vi "4-1.vi"() -> ()   [LabVIEW 2019, in "AoC2022.lvlib"]
uses:
  AoC2022.lvlib
panel:
  out "Array":string[](array[string])
  out "Numeric":i32
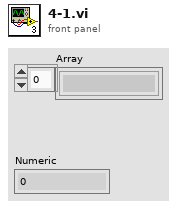
[diagram p1: front panel]
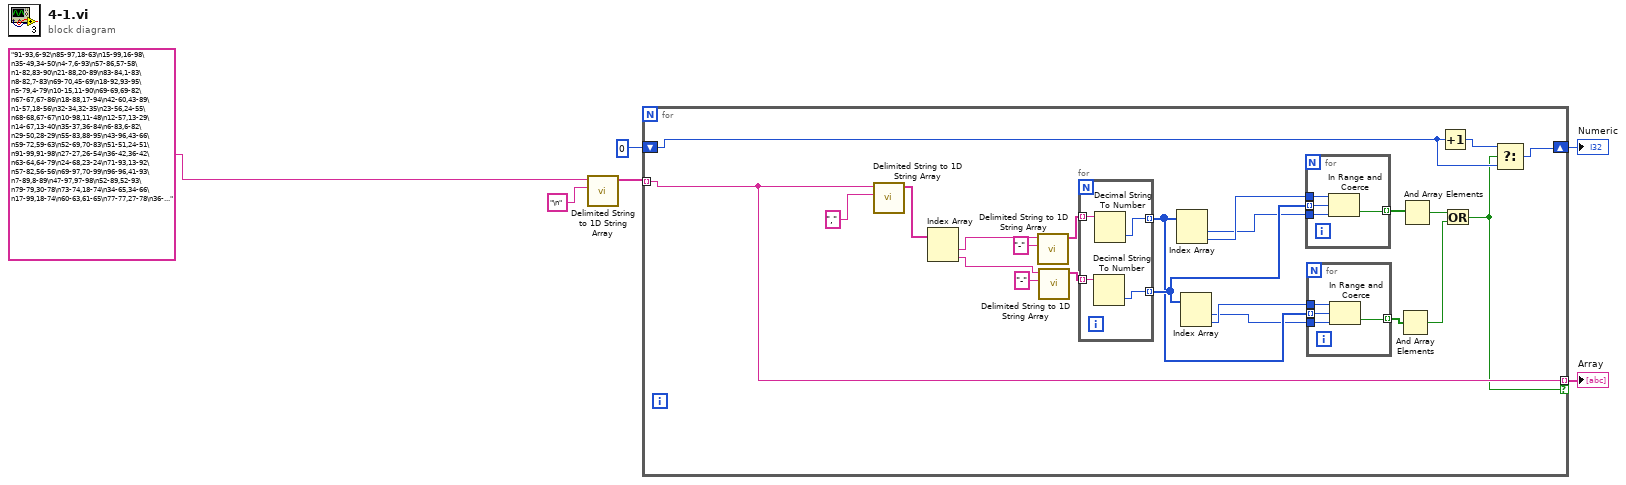
[diagram p0: block diagram]
diagram:
  n1 = call <vilib>:"Delimited String to 1D String Array.vi"("delimiter"="\n", "delimited string"="91-93,6-92\n85-97,18-63\n15-99,16-98\n35-49,34-50\n4-7,6-93\n57-86,57-58\n1-82,83-90\n21-88,20-89\n83-84,1-83\n8-82,7-83\n69-70,45-69\n18-92,93-95\n5-79,4-79\n10-15,11-90\n69-69,69-82\n67-67,67-86\n18-88,17-94\n42-60,43-89\n1-57,18-56\n32-34,32-35\n23-56,24-55\n68-68,67-67\n10-98,11-48\n12-57,13-29\n14-67,13-40\n35-37,36-84\n6-83,6-82\n29-50,28-29\n55-83,88-95\n43-96,43-66\n59-72,59-63\n52-69,70-83\n51-51,24-51\n91-99,91-98\n27-27,26-54\n36-42,36-42\n63-64,64-79\n24-68,23-24\n71-93,13-92\n57-82,56-56\n69-97,70-99\n96-96,41-93\n7-89,8-89\n47-97,97-98\n52-89,52-93\n79-79,30-78\n73-74,18-74\n34-65,34-66\n17-99,18-74\n60-63,61-65\n77-77,27-78\n36-52,51-53\n6-7,7-98\n14-35,36-91\n3-3,5-82\n24-24,25-97\n4-65,3-18\n2-9,10-90\n14-82,15-76\n3-3,3-32\n43-85,43-86\n91-91,23-92\n65-98,10-84\n8-71,9-72\n94-94,6-95\n64-66,65-65\n5-75,4-4\n19-76,20-55\n31-98,32-99\n3-83,3-12\n70-71,21-71\n28-36,37-50\n6-95,5-94\n56-56,56-67\n17-77,25-95\n24-50,25-51\n36-60,60-73\n30-50,48-63\n4-98,5-97\n42-42,42-56\n15-17,16-46\n35-69,36-70\n22-49,22-95\n41-77,36-36\n48-92,47-96\n7-89,6-88\n20-94,20-94\n9-75,73-76\n35-60,35-58\n35-90,35-94\n1-93,1-94\n26-26,26-45\n29-98,28-94\n55-86,45-68\n24-87,25-87\n94-94,17-93\n35-93,36-92\n9-28,9-90\n25-74,26-73\n12-79,11-98\n58-92,57-93\n1-64,2-63\n96-97,7-97\n44-62,62-69\n77-90,6-52\n1-96,96-97\n55-66,54-68\n1-86,1-85\n28-91,28-94\n6-89,5-89\n9-35,9-9\n2-22,1-34\n16-56,54-57\n36-44,44-68\n29-87,11-87\n30-32,31-54\n18-76,10-10\n12-13,13-26\n18-46,17-55\n12-53,13-54\n30-67,31-66\n22-60,22-22\n42-94,42-42\n6-65,66-98\n41-43,42-98\n47-71,48-72\n8-65,7-46\n25-63,6-12\n57-62,24-56\n15-29,14-33\n21-65,20-94\n27-94,28-89\n88-95,5-72\n65-80,64-81\n72-73,39-72\n22-48,21-48\n5-6,13-80\n54-80,55-79\n34-66,31-43\n26-52,51-66\n27-28,15-27\n90-99,89-99\n25-55,26-27\n29-94,29-95\n27-96,96-96\n35-65,65-66\n15-56,63-84\n36-83,35-37\n15-72,15-15\n14-90,15-34\n2-41,4-42\n48-75,47-56\n23-63,63-78\n8-90,5-89\n41-65,12-66\n48-61,54-60\n28-90,29-35\n51-83,85-87\n9-95,9-92\n57-76,57-69\n2-66,2-65\n7-92,11-92\n26-89,88-88\n37-37,37-86\n33-37,36-84\n3-97,99-99\n29-32,29-57\n35-69,5-35\n5-97,5-97\n60-86,44-87\n41-88,98-98\n52-55,53-57\n27-93,28-92\n95-97,50-91\n45-62,45-84\n1-60,2-42\n7-97,98-99\n91-92,18-91\n10-53,11-95\n75-80,77-84\n1-1,1-99\n7-77,27-41\n6-96,96-96\n17-97,17-96\n1-1,1-99\n28-90,29-32\n2-79,12-80\n47-47,10-46\n97-98,2-97\n38-64,38-40\n5-97,4-30\n8-91,7-92\n21-49,20-21\n21-77,20-95\n16-70,15-26\n33-98,32-96\n3-4,8-72\n48-98,2-99\n7-30,8-30\n34-60,33-34\n78-92,34-83\n5-46,5-5\n52-73,35-74\n37-96,97-99\n6-92,5-92\n3-85,3-84\n2-86,2-2\n93-98,72-92\n23-34,22-34\n6-73,5-7\n29-42,29-67\n12-97,11-29\n38-68,38-67\n85-87,81-86\n23-29,30-64\n2-3,3-83\n17-92,18-64\n28-29,29-38\n52-54,53-83\n6-19,6-90\n8-97,79-97\n2-40,2-30\n3-89,4-98\n6-89,1-3\n8-8,8-94\n5-94,4-93\n81-95,81-87\n86-88,87-89\n8-8,9-94\n46-56,46-46\n7-95,32-99\n3-93,2-31\n80-80,1-79\n64-98,63-64\n82-84,14-83\n26-79,26-80\n30-56,57-88\n6-15,49-93\n8-30,4-33\n55-99,13-97\n5-6,6-38\n10-49,12-50\n5-79,78-79\n7-93,6-94\n12-65,64-65\n14-15,15-90\n95-95,48-94\n1-93,3-94\n49-88,88-95\n13-13,13-83\n8-98,97-98\n20-22,21-43\n83-88,84-87\n22-88,21-88\n47-98,35-46\n1-5,6-82\n59-86,65-85\n38-43,40-64\n23-96,22-97\n81-83,67-80\n70-96,70-70\n72-89,62-67\n5-83,6-84\n10-85,2-15\n1-3,2-56\n2-37,37-38\n5-94,4-85\n1-2,3-97\n1-95,97-97\n14-29,15-20\n16-22,29-97\n80-89,89-90\n22-75,21-75\n9-88,6-7\n6-10,11-22\n9-79,9-80\n42-57,18-41\n34-96,96-97\n16-96,17-95\n21-21,22-85\n16-67,15-16\n23-72,60-71\n9-81,9-81\n44-91,45-92\n3-91,4-92\n38-92,69-91\n72-96,2-73\n2-46,1-85\n28-71,28-71\n8-81,7-9\n1-12,1-2\n10-92,3-91\n55-95,96-98\n40-50,41-98\n7-8,8-29\n22-48,23-61\n81-90,25-82\n17-34,17-72\n88-88,5-88\n34-78,34-77\n66-68,67-76\n50-98,49-50\n60-73,6-59\n12-71,12-70\n14-69,68-69\n5-7,6-79\n21-81,21-21\n3-30,4-29\n4-4,6-94\n20-85,19-20\n21-40,22-39\n3-93,2-93\n47-50,50-68\n4-97,5-99\n28-46,27-53\n18-18,17-86\n12-76,77-77\n10-96,11-78\n6-88,4-89\n7-98,7-98\n4-47,3-4\n37-41,38-61\n26-92,26-57\n8-49,14-50\n19-73,18-64\n70-71,3-70\n4-4,4-99\n11-99,62-74\n4-27,4-9\n38-65,38-66\n73-81,79-96\n11-75,10-10\n24-56,55-55\n30-30,31-75\n48-94,49-95\n2-98,3-8\n63-87,62-87\n7-95,73-97\n96-97,15-98\n8-58,57-64\n6-81,80-99\n34-78,78-79\n43-44,44-60\n68-78,78-78\n1-1,3-92\n30-57,53-56\n26-82,26-81\n24-92,24-91\n42-62,43-57\n28-76,77-85\n6-50,6-50\n8-70,9-86\n79-79,32-78\n21-93,27-94\n71-85,65-70\n40-85,41-73\n46-46,47-91\n3-99,4-98\n14-24,13-57\n11-15,17-82\n49-63,39-53\n26-27,19-26\n19-98,18-47\n3-96,3-3\n17-20,16-63\n2-14,2-27\n16-37,13-15\n13-14,14-84\n4-80,3-79\n15-79,14-15\n7-7,8-72\n12-99,99-99\n23-93,24-32\n4-26,3-58\n33-33,38-58\n60-75,59-61\n6-6,6-97\n3-34,2-95\n66-85,66-84\n8-65,9-40\n57-58,58-61\n4-41,5-28\n36-96,35-95\n5-94,1-95\n54-57,56-75\n26-26,26-41\n7-92,7-95\n26-33,5-32\n37-49,38-67\n42-51,52-55\n55-55,31-54\n1-1,1-32\n85-98,9-96\n97-97,77-96\n7-77,6-83\n73-89,72-95\n24-78,27-79\n8-14,3-7\n23-23,23-74\n4-74,3-73\n15-15,17-48\n3-99,3-3\n15-62,15-62\n21-97,6-37\n98-99,64-92\n40-65,41-58\n61-86,1-60\n95-96,23-95\n40-65,39-66\n3-66,2-4\n5-85,6-96\n86-88,85-89\n6-94,82-93\n31-31,32-75\n4-4,3-55\n18-83,19-84\n12-99,11-12\n51-53,49-54\n17-17,18-87\n4-62,61-61\n10-14,14-73\n5-78,6-79\n21-53,22-62\n37-39,38-39\n22-23,23-78\n31-83,35-84\n35-76,36-60\n67-69,68-82\n4-64,29-79\n42-43,52-87\n11-13,12-34\n25-65,70-71\n46-46,46-46\n5-80,3-55\n12-46,10-47\n16-49,1-16\n56-98,32-56\n36-83,37-99\n58-58,53-89\n66-74,8-48\n71-90,34-65\n10-79,1-3\n3-13,4-12\n65-66,66-99\n6-93,5-98\n17-90,18-40\n94-96,15-75\n83-90,99-99\n9-47,10-89\n5-79,6-81\n22-44,16-18\n7-7,7-90\n2-94,1-94\n33-68,24-34\n1-8,12-72\n87-96,73-93\n8-97,97-99\n18-45,19-46\n14-93,13-90\n47-47,48-48\n10-89,11-44\n43-75,76-94\n18-54,17-17\n6-82,7-84\n40-78,78-83\n15-15,16-21\n19-68,50-67\n25-27,30-77\n11-69,10-68\n38-38,48-84\n69-98,68-93\n11-16,17-93\n7-26,27-75\n73-97,73-93\n9-92,8-93\n23-62,62-99\n19-89,19-95\n51-53,15-52\n6-31,30-32\n93-94,10-49\n31-52,30-38\n43-45,44-92\n14-42,13-29\n21-24,22-80\n70-79,24-80\n49-49,49-87\n2-3,2-50\n5-95,6-95\n20-57,16-66\n38-69,68-68\n60-90,91-92\n55-97,94-99\n30-90,30-84\n29-51,30-51\n55-55,42-56\n9-96,8-97\n58-96,58-58\n37-97,98-99\n5-69,5-47\n20-93,21-84\n9-65,1-2\n23-24,24-69\n7-95,8-94\n7-43,8-99\n7-63,4-5\n4-17,4-21\n21-28,27-84\n10-23,10-88\n4-52,4-52\n99-99,89-97\n84-90,1-85\n51-90,99-99\n33-67,53-79\n29-29,2-30\n2-88,1-86\n16-99,3-98\n83-96,82-83\n83-85,20-84\n6-6,7-62\n44-78,58-94\n7-25,7-25\n7-94,8-80\n16-97,15-98\n4-52,51-71\n75-92,49-69\n2-94,2-2\n14-29,15-99\n8-78,8-78\n11-95,12-96\n1-95,1-94\n78-87,11-77\n54-76,54-77\n92-97,90-94\n31-87,32-88\n60-61,2-60\n9-76,10-77\n41-86,2-86\n9-94,9-94\n85-94,9-86\n2-98,98-98\n79-89,58-75\n34-44,33-44\n40-98,39-41\n16-66,15-79\n51-90,90-94\n85-85,86-90\n38-45,34-37\n1-6,5-36\n43-95,43-95\n77-93,66-92\n93-94,8-93\n37-70,36-71\n19-22,22-23\n64-78,63-79\n51-63,7-50\n21-99,20-20\n30-79,30-78\n38-71,32-70\n69-75,69-77\n42-76,41-42\n1-99,2-96\n15-75,15-82\n39-40,40-96\n5-41,42-97\n71-93,70-93\n23-23,23-91\n75-92,79-84\n32-34,33-63\n9-91,76-92\n12-92,11-11\n31-32,8-31\n3-89,2-46\n2-93,2-2\n22-91,22-90\n16-98,5-96\n94-94,4-94\n39-75,39-39\n68-69,3-68\n70-89,70-89\n19-81,19-80\n22-97,23-98\n42-73,42-59\n14-40,14-41\n47-58,46-61\n2-26,3-45\n92-93,44-93\n17-46,18-46\n30-84,53-83\n65-93,94-94\n3-6,6-93\n14-75,32-74\n24-54,23-24\n61-79,47-80\n7-11,16-37\n31-70,30-70\n50-76,51-51\n2-90,89-91\n8-90,7-8\n54-84,61-85\n70-87,71-87\n25-80,7-98\n5-16,4-92\n20-66,21-67\n8-59,7-58\n55-87,30-35\n89-98,24-94\n34-85,34-34\n70-75,17-30\n35-35,36-99\n12-12,11-83\n85-98,86-88\n19-92,16-91\n43-89,17-83\n15-97,15-96\n9-58,9-9\n97-98,5-98\n3-79,99-99\n21-54,20-20\n78-89,77-89\n61-63,20-35\n94-94,37-93\n4-24,3-33\n15-99,16-98\n6-80,6-37\n29-31,30-49\n20-94,21-57\n7-72,7-7\n14-92,14-98\n35-50,50-96\n1-91,2-94\n2-80,1-1\n17-18,18-84\n60-62,34-61\n32-63,31-64\n17-96,18-95\n98-99,8-97\n71-81,81-82\n36-97,35-97\n28-28,27-75\n4-98,3-99\n3-79,19-87\n26-42,25-41\n29-84,22-28\n24-59,60-63\n19-19,19-32\n18-98,18-95\n5-98,6-97\n1-13,46-88\n11-79,11-11\n14-39,15-41\n2-53,6-93\n3-91,2-90\n46-89,45-46\n11-87,10-88\n3-88,3-4\n19-46,47-93\n23-60,22-84\n22-84,21-94\n1-3,18-81\n24-88,10-92\n37-57,38-58\n45-47,46-67\n37-77,36-56\n29-89,29-29\n11-11,11-93\n4-82,57-98\n10-99,10-98\n12-58,12-91\n33-90,34-91\n37-61,37-62\n22-67,7-68\n55-57,38-56\n49-67,67-68\n3-19,20-95\n31-94,94-95\n97-99,7-96\n41-90,40-90\n32-48,31-31\n12-95,2-11\n68-98,16-67\n85-86,42-85\n18-81,17-82\n45-52,44-46\n19-51,18-89\n2-93,94-95\n61-70,61-63\n28-30,29-58\n28-71,71-72\n24-36,29-51\n32-89,74-96\n15-20,13-21\n24-55,23-74\n74-91,92-93\n51-63,50-50\n93-95,95-96\n7-88,6-69\n34-78,88-94\n5-58,5-15\n57-88,87-89\n35-92,36-94\n31-65,32-64\n6-70,5-70\n51-83,51-82\n69-83,69-81\n82-86,61-85\n14-78,78-79\n37-38,40-54\n23-46,22-22\n92-96,93-99\n3-5,4-89\n72-73,15-73\n59-76,74-96\n6-80,2-4\n2-85,3-3\n17-97,20-98\n4-19,20-60\n16-91,17-81\n97-98,12-95\n16-16,16-65\n4-23,3-8\n83-91,19-78\n1-1,1-28\n7-9,8-92\n21-23,22-65\n32-99,32-97\n6-31,6-81\n39-67,39-79\n73-99,42-85\n6-96,5-99\n55-96,39-91\n86-88,9-85\n32-74,33-73\n96-98,13-61\n14-91,91-95\n3-88,2-90\n54-59,60-86\n66-66,66-66\n14-96,13-89\n15-94,69-93\n49-50,49-78\n18-67,18-68\n31-92,30-93\n3-58,4-57\n30-75,30-76\n99-99,70-98\n12-94,93-93\n22-55,23-63\n4-86,59-85\n10-12,13-98\n17-95,17-17\n7-97,67-99\n29-66,43-67\n3-79,1-2\n27-84,18-26\n9-81,8-9\n5-69,1-6\n11-99,12-97\n12-12,14-85\n23-81,24-84\n12-18,35-77\n11-52,12-47\n15-23,69-73\n4-55,2-2\n5-65,65-68\n23-96,24-95\n49-54,49-55\n10-51,9-51\n92-93,68-92\n15-15,17-78\n41-98,40-42\n15-31,14-61\n2-4,4-4\n38-56,40-58\n2-98,11-97\n49-49,50-65\n63-64,64-80\n35-54,3-55\n15-94,16-74\n8-60,16-61\n10-10,9-9\n63-92,63-91\n54-75,54-65\n3-8,11-82\n2-3,3-99\n37-72,37-72\n26-85,25-81\n18-44,17-44\n76-93,62-76\n2-93,3-80\n91-91,90-93\n27-96,27-92\n6-99,5-47\n45-71,45-45\n5-10,6-22\n78-79,77-84\n40-57,39-49\n40-72,41-63\n67-94,67-93\n69-96,54-72\n42-43,41-94\n32-95,31-64\n87-93,18-94\n34-96,35-75\n28-98,98-99\n17-44,16-45\n9-48,8-88\n42-64,42-63\n57-70,58-62\n25-92,18-24\n68-73,67-69\n50-96,14-51\n13-38,12-13\n62-69,61-81\n11-16,29-90\n21-74,21-73\n32-54,33-57\n13-58,13-58\n7-73,7-7\n15-89,14-15\n11-57,11-58\n4-97,3-96\n12-98,11-99\n38-39,37-43\n16-66,15-67\n26-33,27-29\n99-99,71-97\n58-60,57-59\n37-63,44-62\n31-32,32-93\n84-98,87-92\n94-99,76-80\n17-77,76-78\n64-78,45-49\n26-76,25-79\n1-99,99-99\n7-93,7-93\n31-88,91-96\n2-3,5-91\n26-34,35-59\n95-98,63-94\n16-72,17-44\n4-91,4-90\n19-89,20-97\n95-99,1-95\n81-86,81-81\n18-99,75-87\n17-59,18-59\n25-83,25-25\n41-69,40-68\n57-62,57-63\n62-62,51-59\n16-97,15-16\n71-85,11-84\n68-70,49-69\n36-85,37-79\n26-28,26-28\n41-75,37-64\n79-87,79-87\n4-56,3-57\n12-76,13-77\n36-37,7-35\n43-92,29-93\n47-78,47-79\n11-61,11-75\n7-48,7-44\n25-76,24-76\n8-55,55-56\n8-97,7-87\n14-97,99-99\n10-12,11-95\n19-86,18-19\n29-86,13-28\n51-61,50-77\n59-83,59-83\n2-52,1-53\n14-84,15-83\n11-89,11-90\n15-89,16-85\n1-3,5-94\n49-70,69-71\n1-1,3-96\n75-89,75-79\n30-78,31-31\n4-67,4-95\n14-64,15-65\n88-97,9-89\n99-99,7-93\n38-52,39-39\n11-91,11-91\n85-86,14-85\n36-55,14-56\n9-70,70-71\n10-20,76-96\n17-35,35-36\n80-81,21-80\n71-94,17-95\n2-89,14-90\n85-86,39-86\n72-94,71-97\n9-31,8-9\n8-9,9-89\n29-30,29-95\n4-58,5-59\n51-72,50-51\n26-26,26-96\n71-73,50-72\n3-84,1-4\n5-94,95-95\n86-98,85-97\n87-87,34-87\n24-47,25-33\n4-15,15-58\n29-56,56-57\n63-91,32-62\n58-94,58-94\n1-22,2-25\n2-84,2-85\n30-87,29-87\n9-90,9-89\n4-45,5-27\n32-83,31-32\n24-94,23-95\n63-69,63-68\n47-79,47-78\n31-78,31-67\n11-26,6-6\n76-77,40-75\n85-91,22-84\n22-22,22-23\n36-70,36-70\n41-41,41-90\n4-78,2-2\n13-94,12-48\n7-7,20-35\n5-5,4-66\n40-68,50-83\n36-93,35-36\n4-92,42-97\n31-31,20-30\n27-37,28-32\n39-75,40-75\n81-96,80-90\n7-22,8-92\n1-1,3-99\n21-82,22-81\n45-59,28-60\n24-24,24-93\n30-67,68-84\n6-88,6-88\n36-61,8-18\n19-40,39-67\n15-79,16-99\n80-81,80-86\n16-16,17-22\n4-94,3-94\n14-71,13-75\n8-82,7-87\n8-20,9-43\n32-84,31-83\n66-94,13-65\n19-96,22-84\n21-94,22-94\n14-82,50-93\n3-94,1-1\n27-82,33-81\n47-71,48-66\n5-92,12-94\n37-99,14-67\n61-63,5-62\n5-95,4-6\n50-91,25-49\n7-23,22-96\n23-78,24-79\n21-33,22-25\n55-75,9-55\n59-65,41-43\n32-71,32-71\n92-92,10-91\n29-83,17-84\n55-90,90-91\n42-75,41-75\n5-95,5-95\n94-94,67-94\n97-98,35-97\n87-88,60-87\n46-97,47-96\n3-39,40-71\n31-94,30-39\n22-90,21-90\n36-79,36-36\n12-80,12-80\n20-96,19-20\n3-39,4-46\n21-89,99-99\n35-36,34-38\n15-93,22-93\n85-95,86-94\n8-29,7-34\n65-73,67-81\n6-88,83-92") -> ("string array"=w5:string[])  [unwired: 9 in]
  n2 = for {
    tunnel: w5 -> [w8] mode=indexing
    shift-right: [w14] -> w2
    shift-left: 0 -> [w13]
    tunnel: [w8] -> w1 mode=indexing if=w7
    n3 = call <vilib>:"Delimited String to 1D String Array.vi"("delimiter"=",", "delimited string"=w8) -> ("string array"=w28:string[])  [unwired: 9 in]
    n4 = Index Array(array=w28) -> (element #1=w27:string, element #2=w24:string)  [unwired: 2 in]
    n5 = call <vilib>:"Delimited String to 1D String Array.vi"("delimiter"="-", "delimited string"=w27) -> ("string array"=w23:string[])  [unwired: 9 in]
    n6 = call <vilib>:"Delimited String to 1D String Array.vi"("delimiter"="-", "delimited string"=w24) -> ("string array"=w22:string[])  [unwired: 9 in]
    n7 = for {
      tunnel: w23 -> [w41] mode=indexing
      tunnel: w22 -> [w40] mode=indexing
      tunnel: [w39] -> w20 mode=indexing
      tunnel: [w38] -> w21 mode=indexing
      n8 = Decimal String To Number(string=w40) -> (number=w38:i32)  [unwired: 2 in, 1 out]
      n9 = Decimal String To Number(string=w41) -> (number=w39:i32)  [unwired: 2 in, 1 out]
    }
    n10 = Index Array(array=w20) -> (element #1=w11:i32, element #2=w12:i32)  [unwired: 2 in]
    n11 = Index Array(array=w21) -> (element #1=w9:i32, element #2=w10:i32)  [unwired: 2 in]
    n12 = for {
      tunnel: w11 -> [w37]
      tunnel: w12 -> [w36]
      tunnel: w21 -> [w35] mode=indexing
      tunnel: [w34] -> w19 mode=indexing
      n13 = In Range and Coerce(upper limit=w36, x=w35, lower limit=w37) -> (In Range?=w34:bool)  [unwired: 1 out]
    }
    n14 = for {
      tunnel: w9 -> [w33]
      tunnel: w10 -> [w32]
      tunnel: w20 -> [w31] mode=indexing
      tunnel: [w30] -> w18 mode=indexing
      n15 = In Range and Coerce(upper limit=w32, x=w31, lower limit=w33) -> (In Range?=w30:bool)  [unwired: 1 out]
    }
    n16 = And Array Elements(Boolean array=w18) -> (logical AND=w16:bool)
    n17 = And Array Elements(Boolean array=w19) -> (logical AND=w17:bool)
    n18 = Increment(x=w13) -> (x+1=w15:i32)
    n19 = Or(x=w17, y=w16) -> (x .or. y?=w7:bool)
    n20 = Select(t=w15, s=w7, f=w13) -> (s? t:f=w14:i32)
  }
  "Numeric" <- w2
  "Array" <- w1
